vi "Write Data.vi"(8 "error in (no error)":errorcluster, 10 "Data":cluster{"X":dbl, "Y":dbl, "Z":dbl}, 11 "Vec3d Class in":refnum<class "Vec3d.lvclass">) -> (0 "error out":errorcluster, 3 "Vec3d Class out":refnum<class "Vec3d.lvclass">)   [LabVIEW 2022 SP3, in "Vec3d.lvclass"]
uses:
  Vec3d.lvclass
  Vec3d.lvclass/Vec3d.ctl
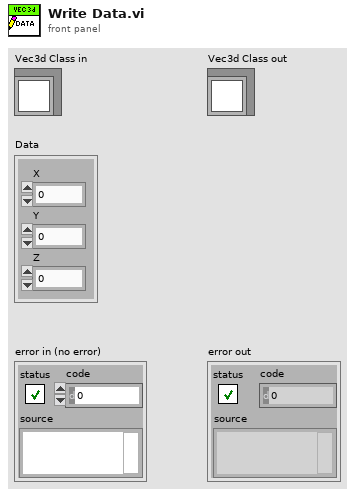
[diagram p1: front panel]
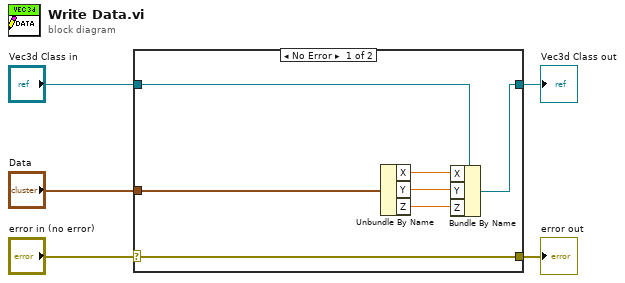
[diagram p0: block diagram]
diagram:
  n1 = case shown="No Error" "error in (no error)" {
    selector: "error in (no error)" -> [w12 w13]
    tunnel: [w12 w13] -> w4
    tunnel: [w10 w14] -> w2
    tunnel: "Vec3d Class in" -> [w11 w14]
    tunnel: "Data" -> [w9 _]
    frame No Error {
      n2 = Unbundle By Name(w9) -> ("X"=w8:dbl, "Y"=w7:dbl, "Z"=w6:dbl)
      n3 = Bundle By Name(cluster=w11, "X"=w8, "Y"=w7, "Z"=w6) -> (w10:refnum<class "Vec3d.lvclass">)
    }
    frame Error {
    }
  }
  "error out" <- w4
  "Vec3d Class out" <- w2
